vi "QX_DisconnectDevice.vi"(8 "Error in":errorcluster, 11 "Devices":refnum<k24>[](array[refnum])) -> (0 "Error out":errorcluster)   [LabVIEW 2016]
doc: "Disconnects all given devices.\n\nDevices: Array of devices to disconnect"
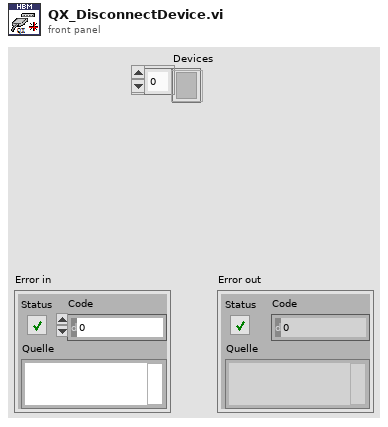
[diagram p1: front panel]
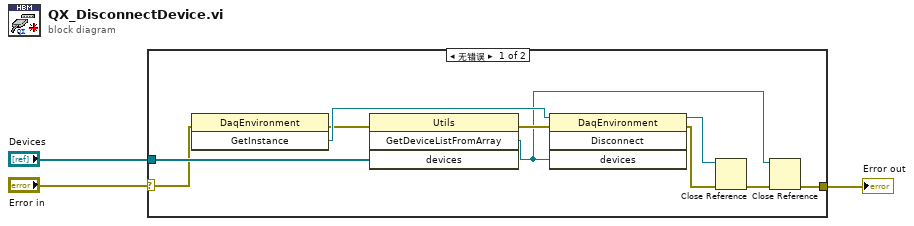
[diagram p0: block diagram]
diagram:
  n1 = case shown="无错误" "Error in" {
    selector: "Error in" -> [w11 w14]
    tunnel: [w4 w14] -> w2
    tunnel: "Devices" -> [w12 _]
    frame No Error {
      n2 = invoke on="Methodenknoten" class="DaqEnvironment" method="GetInstance"(error in=w11) -> (error out=w9:errorcluster, "GetInstance"=w10:refnum<k24>)  [unwired: 2 in, 1 out]
      n3 = invoke on="Methodenknoten" class="Utils" method="GetDeviceListFromArray"(error in=w9, "devices"=w12) -> (error out=w13:errorcluster, "GetDeviceListFromArray"=w5:refnum<k24>)  [unwired: 2 in, 2 out]
      n4 = invoke class="DaqEnvironment" method="Disconnect"(reference=w10, error in=w13, "devices"=w5) -> (reference out=w7:refnum<k24>, error out=w8:errorcluster)  [unwired: 1 in, 2 out]
      n5 = Close Reference(reference=w7, error in (no error)=w8) -> (error out=w6:errorcluster)
      n6 = Close Reference(reference=w5, error in (no error)=w6) -> (error out=w4:errorcluster)
    }
    frame Error {
    }
  }
  "Error out" <- w2
